vi "TabConMain.vi"() -> ()   [LabVIEW 2017]
doc: "This template is for the Queued Message Handler design pattern.\n\nThe Event Handling Loop generates messages based on user interface actions.\n\nThe Message Handling Loop processes messages generated by the Event Handling Loop, or by other messages. The messages are string values, so new messages can be added easily to the Message Cases case structure in the Message Handling Loop. Each message cluster can also provide an optional value for Message Data, which is a variant that can be converted to whatever message-specific data is required."
uses:
  controls/TabConUI Data.ctl
  support/Message Queue/TabConMessage Queue.lvlib
  support/User Event - Stop/TabConUser Event - Stop.lvlib
panel:
  out "Notifications":string
  in  "Chopping Frequency":dbl[unit](knob) scale=200.0..2000.0
  out "Display <Replace Me>":string
  in  "Do Something Else <Replace Me>":bool
  in  "Do Something <Replace Me>":bool
  in  "Stop Button":bool
  # "These controls have associated \"Value Changed\" events configured in the Event Structure on the diagram.\n\nReplace them (and reconfigure the Event Structure) with the controls you need for your application."
  # "This template is for the Queued Message Handler design pattern.\n\nSee the block diagram for more information on how to use this template."
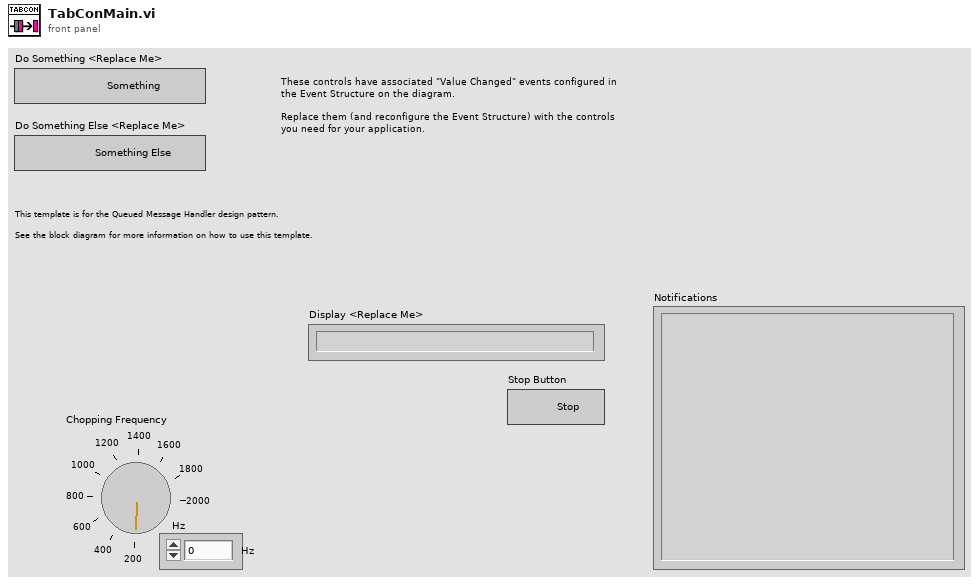
[diagram p1: front panel]
types:
  T1 = typedef "TabConUI Data.ctl" = cluster{"Boolean <Replace Me>":bool, "String <Replace Me>":string, "Numeric <Replace Me>":dbl, "Do Something Ref":refnum<vi>, "Do Something Else Ref":refnum<vi>, "Data Display Ref":refnum<vi>, "Stop Button Ref":refnum<vi>}
  T2 = typedef "TabConMessage Queue.lvlib/All Message Queues.ctl" = cluster{"UI":refnum<queue>}
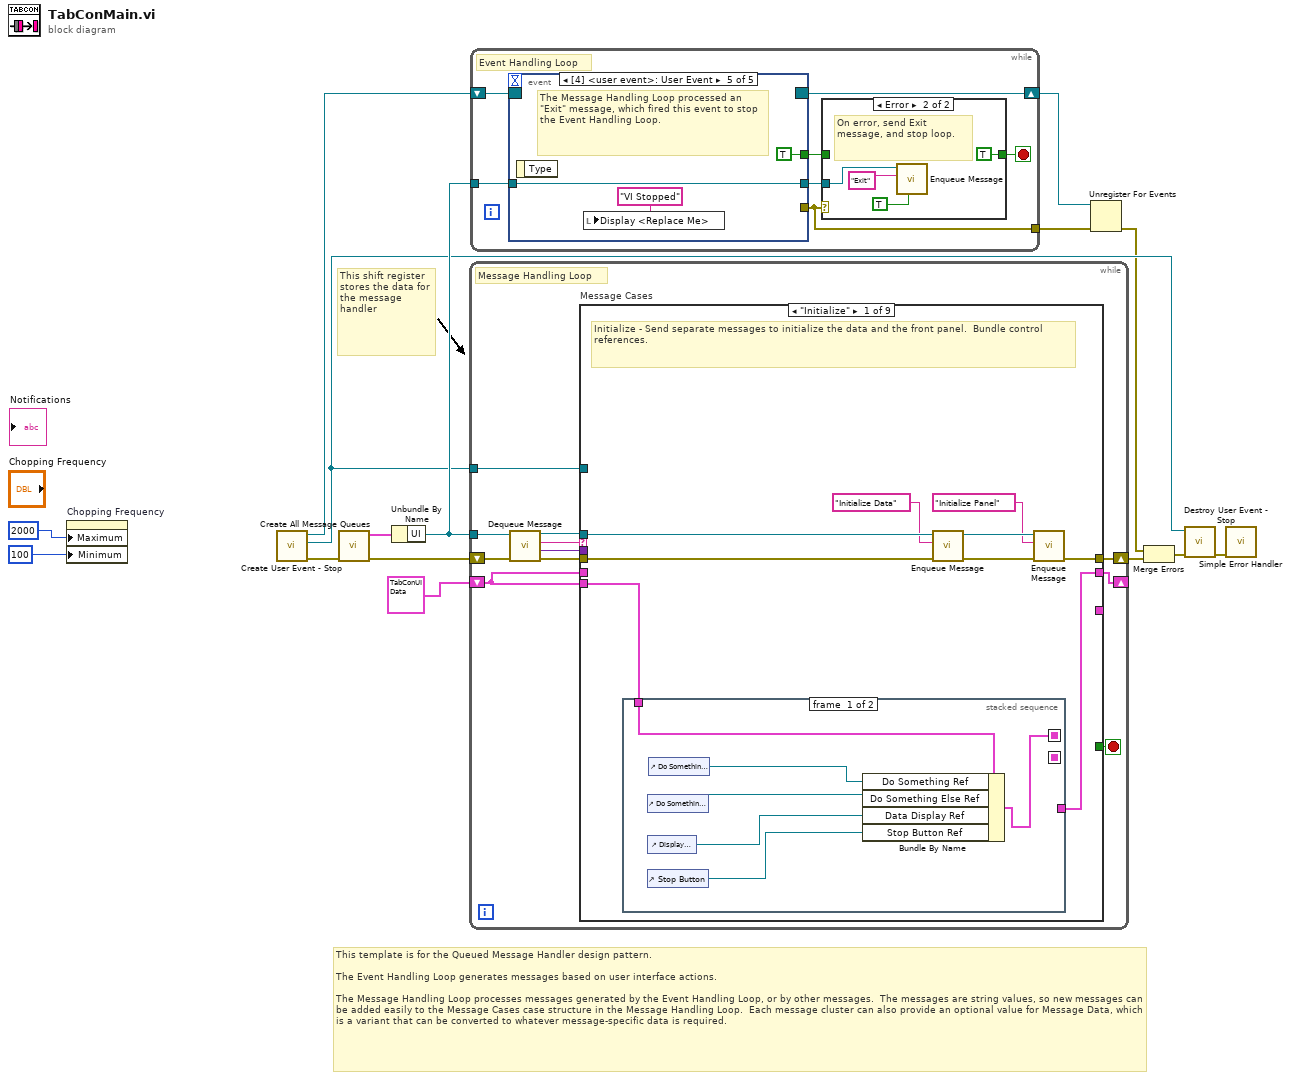
[diagram p0: block diagram]
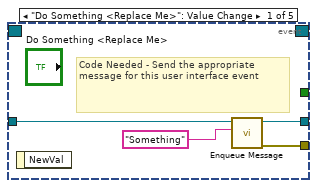
[diagram p3: hidden frame]
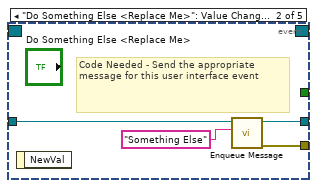
[diagram p4: hidden frame]
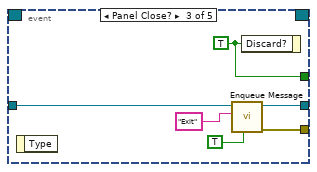
[diagram p5: hidden frame]
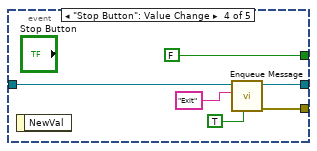
[diagram p6: hidden frame]
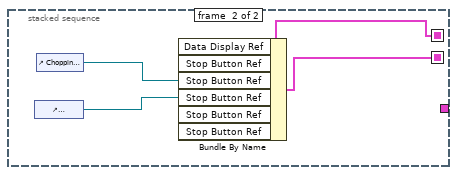
[diagram p7: hidden frame]
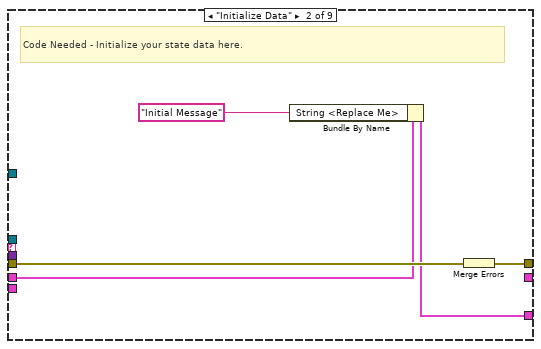
[diagram p8: hidden frame]
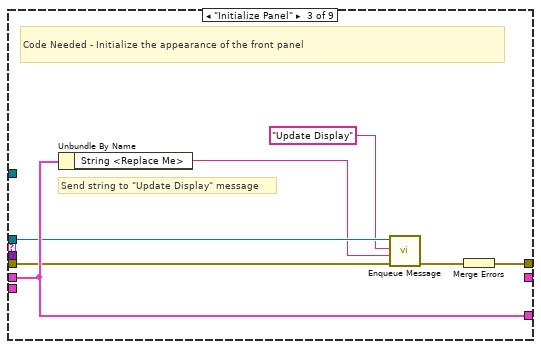
[diagram p9: hidden frame]
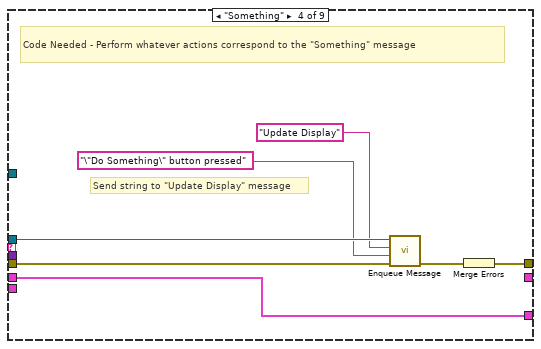
[diagram p10: hidden frame]
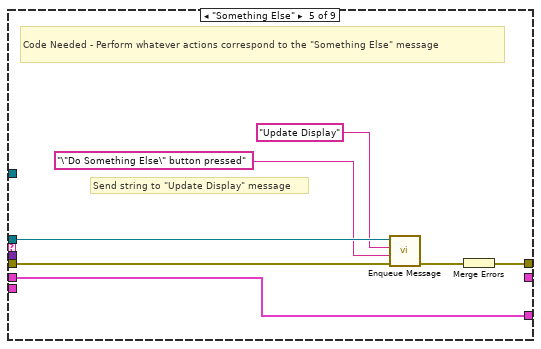
[diagram p11: hidden frame]
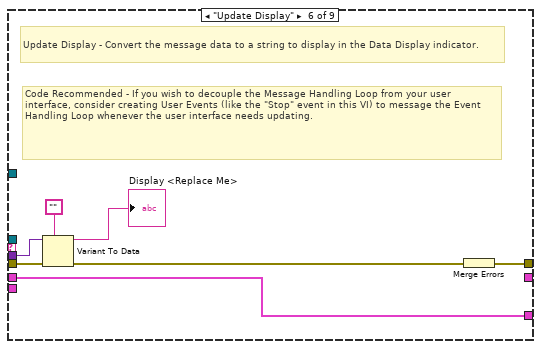
[diagram p12: hidden frame]
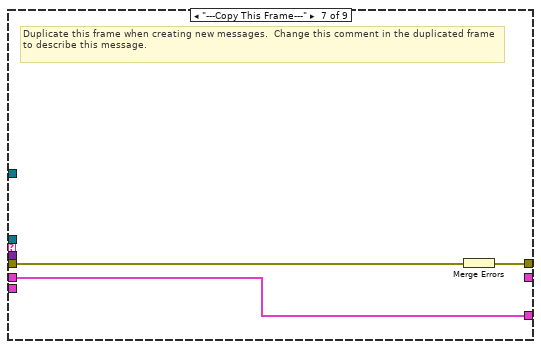
[diagram p13: hidden frame]
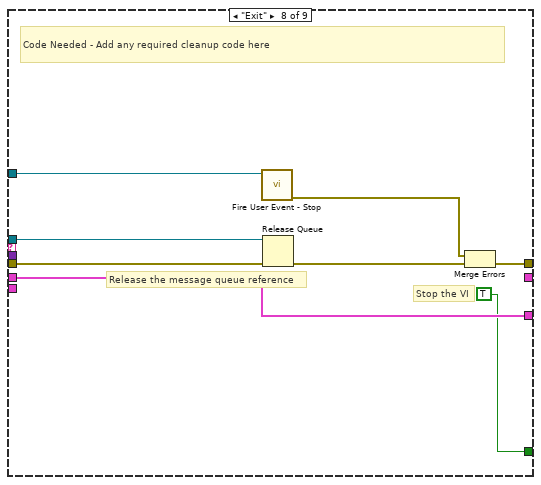
[diagram p14: hidden frame]
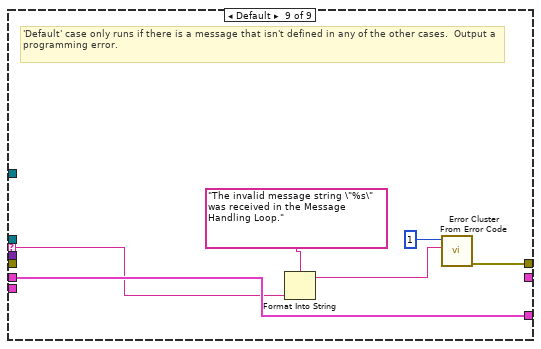
[diagram p15: hidden frame]
diagram:
  # "This template is for the Queued Message Handler design pattern.\n\nThe Event Handling Loop generates messages based on user interface actions.\n\nThe Message Handling Loop processes messages generated by the Event Handling Loop, or by other messages.  The messages are string values, so new messages can be added easily to the Message Cases case structure in the Message Handling Loop.  Each message cluster can also provide an optional value for Message Data, which is a variant that can be converted to whatever message-specific data is required."
  # "This shift register\nstores the data for the message handler"
  n1 = property on="Chopping Frequency" class="Knob (strict)"("Maximum"=2000, "Minimum"=100) -> ()  [unwired: 2 in, 2 out]
  n2 = call "Create User Event - Stop.vi"() -> ("error out"=w10:errorcluster, "User Event - Stop"=w7:refnum<user-event>, "Stop Event Registration Refnum"=w11:refnum<event-registration>)  [unwired: 9 in]
  n3 = call "Create All Message Queues.vi"("error in (no error)"=w10) -> ("error out"=w15:errorcluster, "Message Queues out"=w14:T2)  [unwired: 9 in]
  n4 = Unbundle By Name(w14) -> ("UI"=w12:refnum<queue>)
  n5 = while {
    tunnel: w12 -> [w18]
    shift-right: [w16] -> _
    shift-left: T1 {"Boolean <Replace Me>"=TRUE, "String <Replace Me>"="", "Numeric <Replace Me>"=0.0, "Do Something Ref"=refnum, "Do Something Else Ref"=refnum, "Data Display Ref"=refnum, "Stop Button Ref"=refnum} ("Data Cluster") -> [w17]
    tunnel: w7 -> [w24]
    shift-right: [w25] -> w13
    shift-left: w15 -> [w23]
    stop <- w26 stop-if-true
    # "Message Handling Loop"
    n6 = call "Dequeue Message.vi"("error in (no error)"=w23, "Message Queue"=w18) -> ("error out"=w22:errorcluster, "Message Data"=w20:variant, "Message"=w21:string, "dup Message Queue"=w19:refnum<queue>)  [unwired: 6 in]
    n7 = case "Message Cases" shown="\"Initialize\"" w21 {
      selector: w21 -> [_ _ _ _ _ _ _ _ w93]
      tunnel: w19 -> [w31 _ w54 w60 w67 _ _ w89 _]
      tunnel: w22 -> [w34 w50 w55 w62 w69 w76 w81 w84 _]
      tunnel: [w35 w46 w56 w63 w70 w77 w79 w85 w91] -> w25
      tunnel: w17 -> [_ w49 w57 w64 w71 w78 w80 w88 w95]
      tunnel: [_ w48 w57 w64 w71 w78 w80 w88 w95] -> _
      tunnel: [_ _ _ _ _ _ _ TRUE _] -> w26
      tunnel: w20 -> [_ _ _ _ _ w75 _ _ _]
      tunnel: w24 -> [_ _ _ _ _ _ _ w83 _]
      tunnel: w17 -> [w28 _ _ _ _ _ _ _ _]
      tunnel: [w27 _ _ _ _ _ _ _ _] -> w16
      frame "Initialize" {
        # "Initialize - Send separate messages to initialize the data and the front panel.  Bundle control references."
        n8 = stacked-sequence {
          seq-local: [w36 _] -> [_ w45]
          seq-local: [_ w42] -> [_ _]
          tunnel: w28 -> [w37 _]
          tunnel: [_ _] -> w27
          frame #0 {
            n9 = control-ref of="Do Something Else <Replace Me>"() -> (w40:refnum<vi>)
            n10 = control-ref of="Display <Replace Me>"() -> (w39:refnum<vi>)
            n11 = control-ref of="Stop Button"() -> (w38:refnum<vi>)
            n12 = control-ref of="Do Something <Replace Me>"() -> (w41:refnum<vi>)
            n13 = Bundle By Name(cluster=w37, "Do Something Ref"=w41, "Do Something Else Ref"=w40, "Data Display Ref"=w39, "Stop Button Ref"=w38) -> (w36:T1)
          }
          frame #1 {
            n14 = control-ref of="Notifications"() -> (w43:refnum<vi>)
            n15 = control-ref of="Chopping Frequency"() -> (w44:refnum<vi>)
            n16 = Bundle By Name(cluster=w45, "Stop Button Ref"=w44, "Stop Button Ref"=w43) -> (w42:T1)  [unwired: 4 in]
          }
        }
        n17 = call "Enqueue Message.vi"("error in (no error)"=w34, "Message"="Initialize Data", "Message Queue"=w31) -> ("error out"=w33:errorcluster, "dup Message Queue"=w32:refnum<queue>)  [unwired: 7 in]
        n18 = call "Enqueue Message.vi"("error in (no error)"=w33, "Message"="Initialize Panel", "Message Queue"=w32) -> ("error out"=w35:errorcluster)  [unwired: 7 in, 1 out]
      }
      frame "Initialize Data" {
        # "Code Needed - Initialize your state data here."
        n19 = Bundle By Name(cluster=w49, "String <Replace Me>"="Initial Message" ("Initial Message")) -> (w48:T1)
        n20 = Merge Errors(w50) -> (w46:errorcluster)
      }
      frame "Initialize Panel" {
        # "Send string to \"Update Display\" message"
        # "Code Needed - Initialize the appearance of the front panel"
        n21 = Unbundle By Name(w57) -> ("String <Replace Me>"=w51:string)
        n22 = call "Enqueue Message.vi"("error in (no error)"=w55, "Message Data"=w51, "Message"="Update Display", "Message Queue"=w54) -> ("error out"=w53:errorcluster)  [unwired: 6 in, 1 out]
        n23 = Merge Errors(w53) -> (w56:errorcluster)
      }
      frame "Something" {
        # "Send string to \"Update Display\" message"
        # "Code Needed - Perform whatever actions correspond to the \"Something\" message"
        n24 = call "Enqueue Message.vi"("error in (no error)"=w62, "Message Data"="\"Do Something\" button pressed" ("\"Do Something\" button pressed"), "Message"="Update Display", "Message Queue"=w60) -> ("error out"=w61:errorcluster)  [unwired: 6 in, 1 out]
        n25 = Merge Errors(w61) -> (w63:errorcluster)
      }
      frame "Something Else" {
        # "Send string to \"Update Display\" message"
        # "Code Needed - Perform whatever actions correspond to the \"Something Else\" message"
        n26 = call "Enqueue Message.vi"("error in (no error)"=w69, "Message Data"="\"Do Something Else\" button pressed" ("\"Do Something Else\" button pressed"), "Message"="Update Display", "Message Queue"=w67) -> ("error out"=w68:errorcluster)  [unwired: 6 in, 1 out]
        n27 = Merge Errors(w68) -> (w70:errorcluster)
      }
      frame "Update Display" {
        # "Code Recommended - If you wish to decouple the Message Handling Loop from your user interface, consider creating User Events (like the \"Stop\" event in this VI) to message the Event Handling Loop whenever the user interface needs updating."
        # "Update Display - Convert the message data to a string to display in the Data Display indicator."
        n28 = Variant To Data(error in=w76, type="", Variant=w75) -> (data=→"Display <Replace Me>":string, error out=w73:errorcluster)
        n29 = Merge Errors(w73) -> (w77:errorcluster)
      }
      frame "---Copy This Frame---" {
        # "Duplicate this frame when creating new messages.  Change this comment in the duplicated frame to describe this message."
        n30 = Merge Errors(w81) -> (w79:errorcluster)
      }
      frame "Exit" {
        # "Stop the VI"
        # "Release the message queue reference"
        # "Code Needed - Add any required cleanup code here"
        n31 = call "Fire User Event - Stop.vi"("User Event - Stop"=w83) -> ("error out"=w82:errorcluster)  [unwired: 10 in]
        n32 = Release Queue(queue=w89, error in (no error)=w84) -> (error out=w86:errorcluster)  [unwired: 1 in, 2 out]
        n33 = Merge Errors(w82, w86) -> (w85:errorcluster)
      }
      frame Default {
        # "'Default' case only runs if there is a message that isn't defined in any of the other cases.  Output a programming error."
        n34 = Format Into String(format string="The invalid message string \"%s\" was received in the Message Handling Loop." ("Unknown Message Error Text"), w93) -> (resulting string=w90:string)  [unwired: 2 in, 1 out]
        n35 = call <vilib>:"Error Cluster From Error Code.vi"("error message (\"\")"=w90, "error code (0)"=1) -> ("error out"=w91:errorcluster)  [unwired: 7 in]
      }
    }
  }
  n36 = while {
    tunnel: w12 -> [w102]
    tunnel: [w98] -> w5
    shift-right: [w96] -> w4
    shift-left: w11 -> [w97]
    stop <- w100 stop-if-true
    # "Event Handling Loop"
    n37 = event shown="[4] <user event>: User Event" {
      selector: w97 -> [_ _ _ _ _]
      dyn-events: [_ _ _ _ _] -> w96
      timeout: _ -> [_ _ _ _ _]
      tunnel: [_ _ w121 FALSE ("Discard?") TRUE ("Discard?")] -> w101
      tunnel: w102 -> [w111 w115 w120 w127 w130]
      tunnel: [w110 w113 w119 w126 _] -> w98
      tunnel: [w109 w114 w118 w124 w130] -> w99
      event "Do Something <Replace Me>": Value Change {
        # "Code Needed - Send the appropriate message for this user interface event"
        n38 = event-data() -> ()  [unwired: 1 in, 1 out]
        n39 = call "Enqueue Message.vi"("Message"="Something", "Message Queue"=w111) -> ("error out"=w110:errorcluster, "dup Message Queue"=w109:refnum<queue>)  [unwired: 8 in]
      }
      event "Do Something Else <Replace Me>": Value Change {
        # "Code Needed - Send the appropriate message for this user interface event"
        n40 = event-data() -> ()  [unwired: 1 in, 1 out]
        n41 = call "Enqueue Message.vi"("Message"="Something Else", "Message Queue"=w115) -> ("error out"=w113:errorcluster, "dup Message Queue"=w114:refnum<queue>)  [unwired: 8 in]
      }
      event Panel Close? {
        w121 = TRUE ("Discard?")
        n42 = event-data() -> ()  [unwired: 1 in, 1 out]
        n43 = call "Enqueue Message.vi"("Priority Message? (F)"=TRUE, "Message"="Exit", "Message Queue"=w120) -> ("error out"=w119:errorcluster, "dup Message Queue"=w118:refnum<queue>)  [unwired: 7 in]
        n44 = event-data("Discard?"=w121) -> ()  [unwired: 1 in, 1 out]
      }
      event "Stop Button": Value Change {
        n45 = event-data() -> ()  [unwired: 1 in, 1 out]
        n46 = call "Enqueue Message.vi"("Priority Message? (F)"=TRUE, "Message"="Exit", "Message Queue"=w127) -> ("error out"=w126:errorcluster, "dup Message Queue"=w124:refnum<queue>)  [unwired: 7 in]
      }
      event User Event {
        # "The Message Handling Loop processed an \"Exit\" message, which fired this event to stop the Event Handling Loop."
        n47 = event-data() -> ()  [unwired: 1 in, 1 out]
        n48 = local write "Display <Replace Me>"("VI Stopped" ("VI Stopped")) -> ()
      }
    }
    n49 = case shown="Error" w98 {
      tunnel: [w103 TRUE ("Discard?")] -> w100
      tunnel: w101 -> [w103 _]
      tunnel: w99 -> [_ w106]
      frame No Error {
      }
      frame Error {
        # "On error, send Exit message, and stop loop."
        n50 = call "Enqueue Message.vi"("Priority Message? (F)"=TRUE, "Message"="Exit", "Message Queue"=w106) -> ()  [unwired: 7 in, 2 out]
      }
    }
  }
  n51 = Unregister For Events(event registration refnum=w4, error in=w5) -> (error out=w6:errorcluster)
  n52 = Merge Errors(w6, w13) -> (w8:errorcluster)
  n53 = call "Destroy User Event - Stop.vi"("error in (no error)"=w8, "User Event - Stop"=w7) -> ("error out"=w9:errorcluster)  [unwired: 9 in]
  n54 = call <vilib>:"Simple Error Handler.vi"("error in (no error)"=w9) -> ()  [unwired: 4 in, 5 out]
